vi "XNET Clear.vi"(0 "session in":refnum<k21>, 11 "error in (no error)":errorcluster) -> (15 "error out":errorcluster)   [LabVIEW 2018]
doc: "Clears (closes) the XNET session."
uses:
  nixlvapi.dll
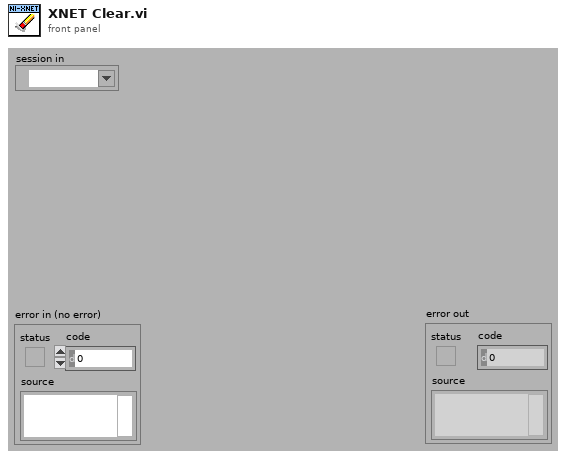
[diagram p1: front panel]
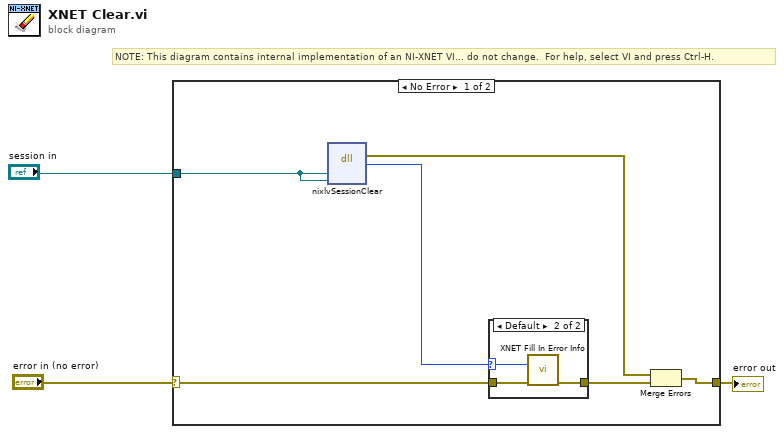
[diagram p0: block diagram]
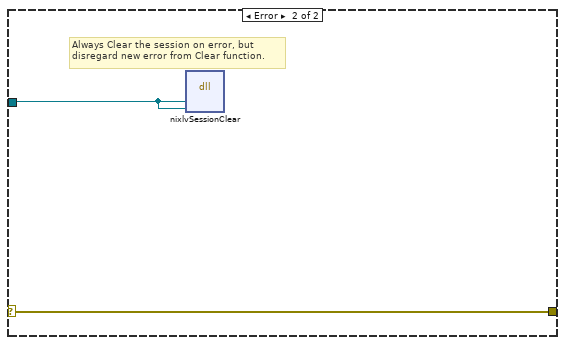
[diagram p3: hidden frame]
diagram:
  # "NOTE: This diagram contains internal implementation of an NI-XNET VI... do not change.  For help, select VI and press Ctrl-H."
  n1 = case shown="No Error" "error in (no error)" {
    selector: "error in (no error)" -> [w9 w15]
    tunnel: "session in" -> [w6 w14]
    tunnel: [w5 w15] -> w3
    frame No Error {
      # "NOTE: This diagram contains internal implementation of an NI-XNET VI... do not change.  For help, select VI and press Ctrl-H."
      n2 = dll-call lib="nixlvapi.*" fn="nixlvSessionClear" ("nilvxaiu.dll:lvxenSessionClear")("Reference"=w6, "RefObjPtr"=w6) -> (error out=w4:errorcluster, "return type"=w7:i32)  [unwired: 4 in, 2 out]
      n3 = case shown="Default" w7 {
        selector: w7 -> [_ w11]
        tunnel: w9 -> [w10 w12]
        tunnel: [w10 w13] -> w8
        frame 0 {
        }
        frame Default {
          n4 = call "XNET Fill In Error Info.vi"("status code"=w11, "error in"=w12) -> ("error out"=w13:errorcluster)  [unwired: 13 out]
        }
      }
      n5 = Merge Errors(w4, w8) -> (w5:errorcluster)
    }
    frame Error {
      # "Always Clear the session on error, but\ndisregard new error from Clear function."
      n6 = dll-call lib="nixlvapi.*" fn="nixlvSessionClear" ("nilvxaiu.dll:lvxenSessionClear")("Reference"=w14, "RefObjPtr"=w14) -> ()  [unwired: 4 in, 4 out]
    }
  }
  "error out" <- w3
